vi "Action Engine Shutdown.vi"(7 "Shutdown":enum16{"Write", "Read"}(ring), 10 "error in (no error)":errorcluster, 11 "Shutdown (True to Shutdown)":bool) -> (2 "error out":errorcluster, 3 "Shutdown":bool)   [LabVIEW 2011]
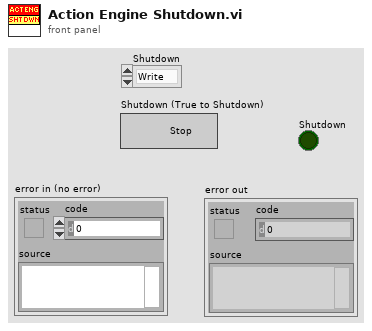
[diagram p1: front panel]
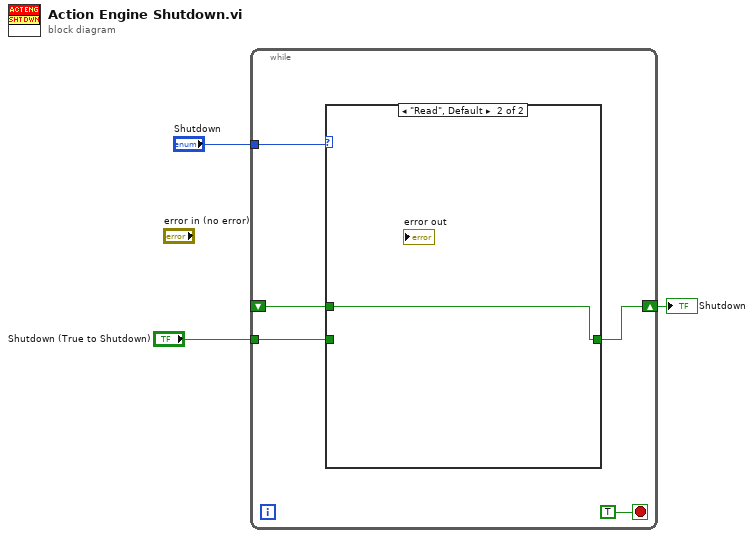
[diagram p0: block diagram]
diagram:
  n1 = while {
    tunnel: "Shutdown (True to Shutdown)" -> [w7]
    tunnel: "Shutdown" -> [w5]
    shift-right: [w6] -> w1
    shift-left: _ -> [w4]
    stop <- TRUE stop-if-true
    n2 = case shown="\"Read\", Default" w5 {
      tunnel: w7 -> [w9 _]
      tunnel: [w9 w10] -> w6
      tunnel: w4 -> [_ w10]
      frame "Write" {
      }
      frame "Read", Default {
      }
    }
  }
  "Shutdown" <- w1
